vi "Get Path Data.vi"(8 "error in":errorcluster, 11 "Path":path) -> (0 "error out":errorcluster, 3 "Path stuff":T4 {"output cluster"."Limits"."StoopidFast (fps)" min=0.0; "output cluster"."Limits"."Jerk (fps^3)" min=0.0 step=1.0; "output cluster"."Limits"."Accel (fps^2)" min=0.0; "output cluster"."Limits"."Velocity (fps)" min=0.0})   [LabVIEW 2019]
uses:
  Single Cmd Info.ctl
  <vilib>/picture/picture.llb/imagedata.ctl
  types/Limits.ctl
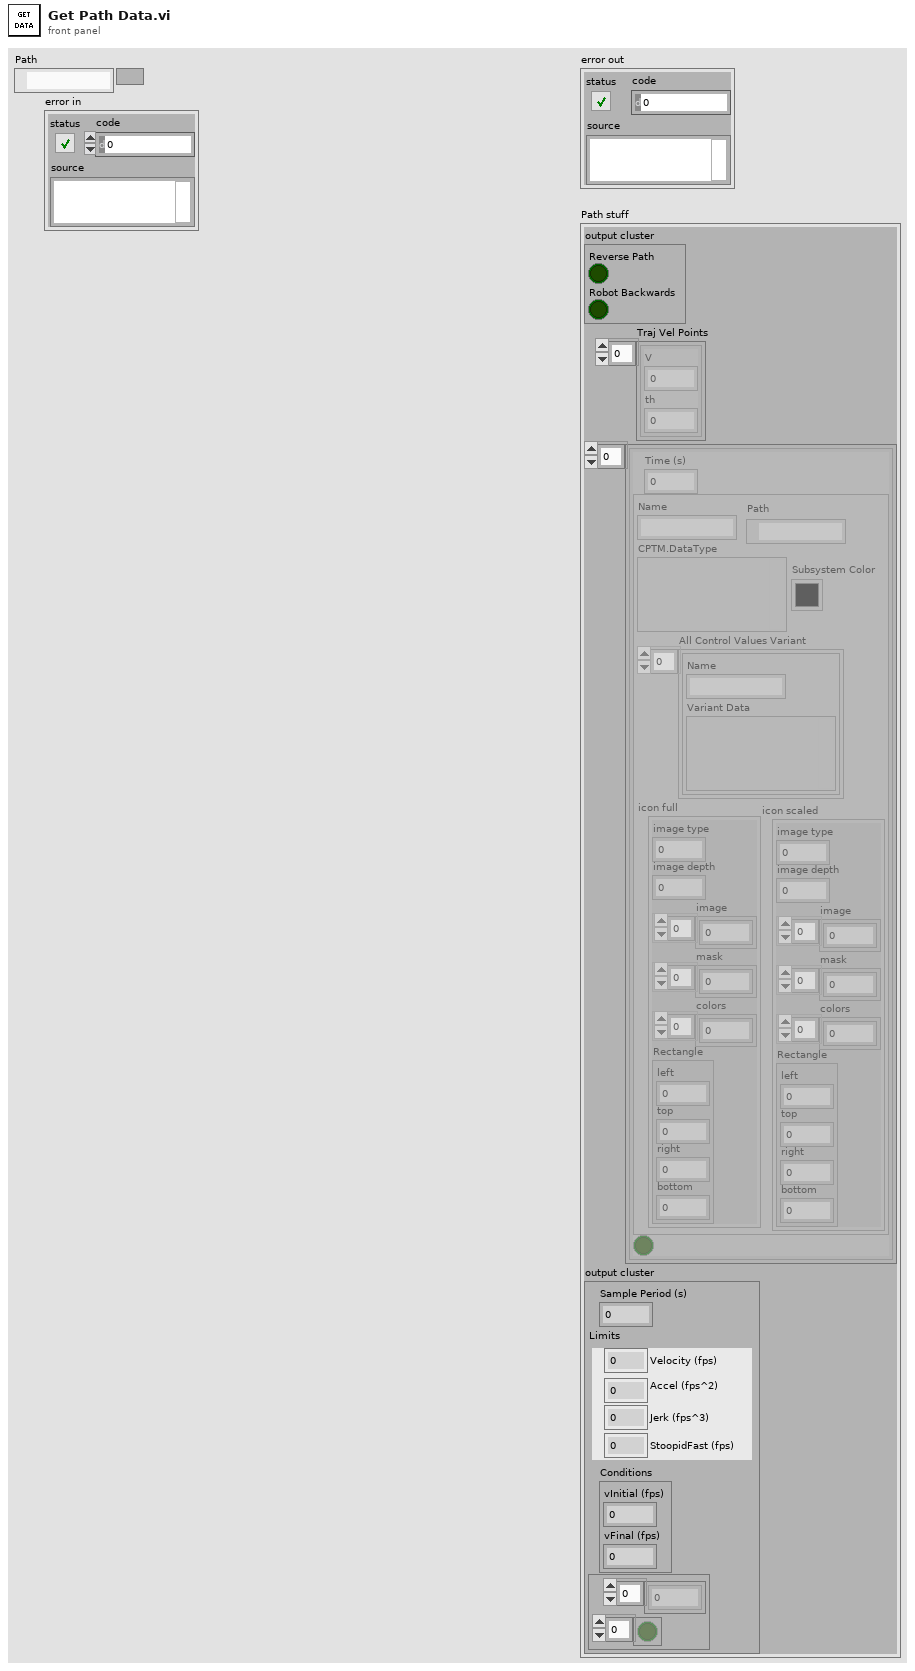
[diagram p1: front panel]
types:
  T1 = typedef "Single Cmd Info.ctl" = cluster{"Name":string, "CPTM.DataType":variant, "All Control Values Variant":cluster{"Name":string, "Variant Data":variant}[], "icon full":T2, "icon scaled":T2, "Path":path, "Subsystem Color":u32}
  T2 = typedef "imagedata.ctl" = cluster{"image type":i32, "image depth":i32, "image":u8[], "mask":u8[], "colors":u32[], "Rectangle":cluster{"left":i16, "top":i16, "right":i16, "bottom":i16}}
  T3 = typedef "Limits.ctl" = cluster{"Velocity (fps)":dbl, "Accel (fps^2)":dbl, "Jerk (fps^3)":dbl, "StoopidFast (fps)":dbl}
  T4 = cluster{"output cluster":cluster{"Reverse Path":bool, "Robot Backwards":bool}, "Traj Vel Points":cluster{"V":dbl, "th":dbl}[], cluster{"Time (s)":dbl, T1, bool}[], "output cluster":cluster{"Sample Period (s)":dbl, "Limits":T3, "Conditions":cluster{"vInitial (fps)":dbl, "vFinal (fps)":dbl}, cluster{dbl[], bool[]}}}
  T5 = cluster{"Segment Name":string, "Type":enum16{"Accel Straight", "Const Straight", "Blend", "Circle"}, "Traj Pos Points":cluster{"x":dbl, "y":dbl, "th":dbl}[], "Traj Vel Points":cluster{"V":dbl, "th":dbl}[], "Accel Index":i32, "Decel Index":i32}[]
  T6 = cluster{"Path Backwards":bool, "Robot Backwards":bool}
  T7 = cluster{"Sample Period (s)":dbl, "Limits":cluster{"Velocity (fps)":dbl, "Acceleration (fps^2)":dbl, "Jerk (fps^3)":dbl}, "Conditions":cluster{"vInitial (fps)":dbl, "vFinal (fps)":dbl}, "Angular Accelerations":cluster{"Angular \nAccelerations":dbl[], "Override Limits?":bool[]}}
  T8 = cluster{"Sample Period (s)":dbl, "Limits":T3, "Conditions":cluster{"vInitial (fps)":dbl, "vFinal (fps)":dbl}, cluster{dbl[], bool[]}}
  T9 = cluster{"Reverse Path":bool, "Robot Backwards":bool}
  T10 = cluster{"Velocity (fps)":dbl, "Acceleration (fps^2)":dbl, "Jerk (fps^3)":dbl}
  T11 = cluster{"vInitial (fps)":dbl, "vFinal (fps)":dbl}
  T12 = cluster{"Angular \nAccelerations":dbl[], "Override Limits?":bool[]}
  T13 = cluster{"Velocity (fps)":dbl, "Acceleration (fps^2)":dbl, "Jerk (fps^3)":dbl, dbl}
  T14 = cluster{"Sample Period (s)":dbl, cluster{"Velocity (fps)":dbl, "Acceleration (fps^2)":dbl, "Jerk (fps^3)":dbl, dbl}, "Conditions":cluster{"vInitial (fps)":dbl, "vFinal (fps)":dbl}, "Angular Accelerations":cluster{"Angular \nAccelerations":dbl[], "Override Limits?":bool[]}}
  T15 = cluster{"Cluster":cluster{"Path Backwards":bool, "Robot Backwards":bool}, "Traj Vel Points":cluster{"V":dbl, "th":dbl}[], cluster{"Time (s)":dbl, T1, bool}[], cluster{"Sample Period (s)":dbl, cluster{"Velocity (fps)":dbl, "Acceleration (fps^2)":dbl, "Jerk (fps^3)":dbl, dbl}, "Conditions":cluster{"vInitial (fps)":dbl, "vFinal (fps)":dbl}, "Angular Accelerations":cluster{"Angular \nAccelerations":dbl[], "Override Limits?":bool[]}}}
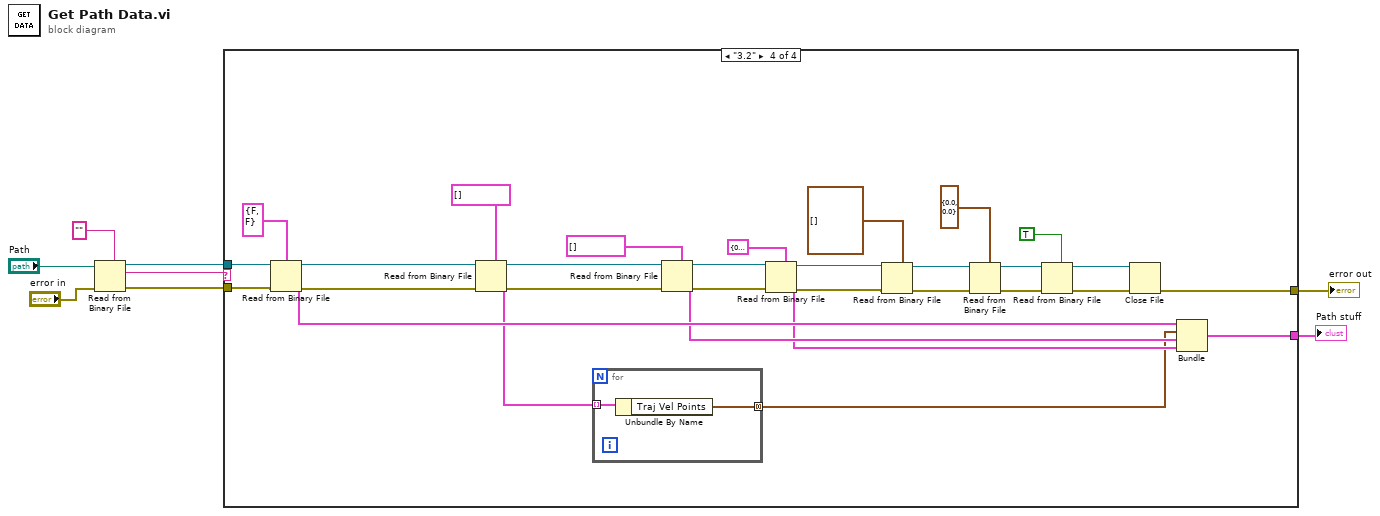
[diagram p0: block diagram]
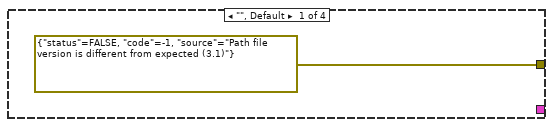
[diagram p2: hidden frame]
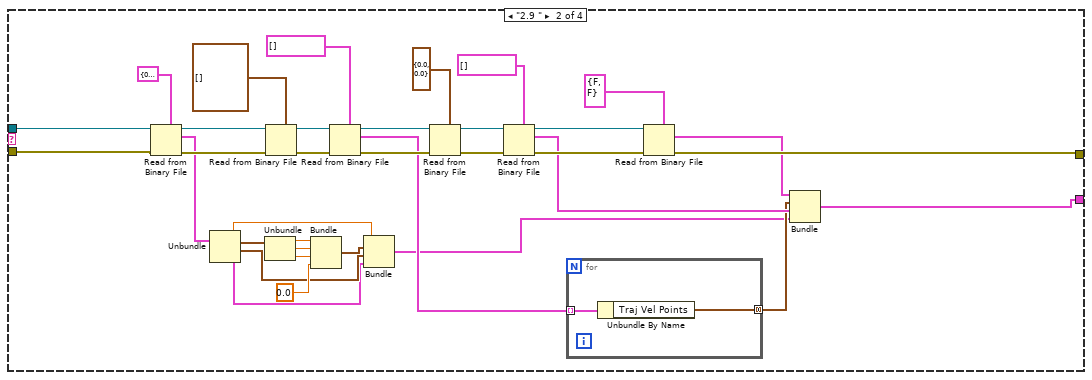
[diagram p3: hidden frame]
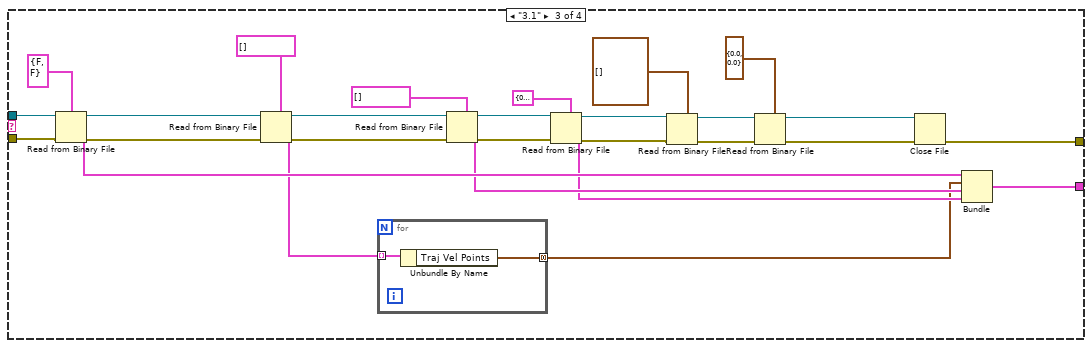
[diagram p4: hidden frame]
diagram:
  n1 = Read from Binary File(5:"", 8:"error in", 11:"Path") -> (0:w4:errorcluster, 2:w2:string, 3:w6:refnum<file>)  [unwired: 3 in, 1 out]
  n2 = case shown="\"3.2\"" w2 {
    tunnel: w6 -> [_ w37 w73 w105]
    tunnel: w4 -> [_ w32 w65 w97]
    tunnel: [errorcluster {"status"=FALSE, "code"=-1, "source"="Path file version is different from expected (3.1)"} ("error out") w26 w53 w87] -> w3
    tunnel: [_ w10 w47 w81] -> w1
    frame "", Default {
    }
    frame "2.9 " {
      n3 = Read from Binary File(5:T7 {"Sample Period (s)"=0.0, "Limits"={"Velocity (fps)"=0.0, "Acceleration (fps^2)"=0.0, "Jerk (fps^3)"=0.0}, "Conditions"={"vInitial (fps)"=0.0, "vFinal (fps)"=0.0}, "Angular Accelerations"={"Angular \nAccelerations"=[], "Override Limits?"=[]}}, 8:w32, 11:w37) -> (0:w31:errorcluster, 2:w21:T7, 3:w40:refnum<file>)  [unwired: 3 in, 1 out]
      n4 = Unbundle(w21) -> ("Sample Period (s)"=w15:dbl, "Limits"=w20:T10, "Conditions"=w13:T11, "Angular Accelerations"=w12:T12)
      n5 = Unbundle(w20) -> ("Velocity (fps)"=w19:dbl, "Acceleration (fps^2)"=w18:dbl, "Jerk (fps^3)"=w17:dbl)
      n6 = Read from Binary File(5:cluster{"x":dbl, "y":dbl, "th":dbl}[] [] ("Points"), 8:w31, 11:w40) -> (0:w30:errorcluster, 3:w41:refnum<file>)  [unwired: 3 in, 2 out]
      n7 = Bundle("Velocity (fps)"=w19, "Acceleration (fps^2)"=w18, "Jerk (fps^3)"=w17, 0.0) -> (w14:T13)  [unwired: 1 in]
      n8 = Read from Binary File(5:T5 [] ("Trajectory Data"), 8:w30, 11:w41) -> (0:w29:errorcluster, 2:w23:T5, 3:w42:refnum<file>)  [unwired: 3 in, 1 out]
      n9 = Bundle("Sample Period (s)"=w15, w14, "Conditions"=w13, "Angular Accelerations"=w12) -> (w11:T14)  [unwired: 1 in]
      n10 = Read from Binary File(5:cluster{"Time (s)":dbl, "Distance (ft)":dbl} {"Time (s)"=0.0, "Distance (ft)"=0.0}, 8:w29, 11:w42) -> (0:w28:errorcluster, 3:w43:refnum<file>)  [unwired: 3 in, 2 out]
      n11 = Read from Binary File(5:cluster{"Time (s)":dbl, T1, bool}[] [], 8:w28, 11:w43) -> (0:w27:errorcluster, 2:w24:cluster{"Time (s)":dbl, T1, bool}[], 3:w44:refnum<file>)  [unwired: 3 in, 1 out]
      n12 = for {
        tunnel: w23 -> [w46] mode=indexing
        tunnel: [w45] -> w22 mode=concatenating
        n13 = Unbundle By Name(w46) -> ("Traj Vel Points"=w45:cluster{"V":dbl, "th":dbl}[])
      }
      n14 = Read from Binary File(5:T6 {"Path Backwards"=FALSE, "Robot Backwards"=FALSE} ("Cluster"), 8:w27, 11:w44) -> (0:w26:errorcluster, 2:w25:T6)  [unwired: 3 in, 2 out]
      n15 = Bundle("Cluster"=w25, "Traj Vel Points"=w22, w24, w11) -> (w10:T15)  [unwired: 1 in]
    }
    frame "3.1" {
      n16 = Read from Binary File(5:T9 {"Reverse Path"=FALSE, "Robot Backwards"=FALSE} ("output cluster"), 8:w65, 11:w73) -> (0:w64:errorcluster, 2:w52:T9, 3:w71:refnum<file>)  [unwired: 3 in, 1 out]
      n17 = Read from Binary File(5:T5 [] ("Trajectory Data"), 8:w64, 11:w71) -> (0:w63:errorcluster, 2:w49:T5, 3:w69:refnum<file>)  [unwired: 3 in, 1 out]
      n18 = for {
        tunnel: w49 -> [w75] mode=indexing
        tunnel: [w74] -> w48 mode=concatenating
        n19 = Unbundle By Name(w75) -> ("Traj Vel Points"=w74:cluster{"V":dbl, "th":dbl}[])
      }
      n20 = Read from Binary File(5:cluster{"Time (s)":dbl, T1, bool}[] [], 8:w63, 11:w69) -> (0:w62:errorcluster, 2:w51:cluster{"Time (s)":dbl, T1, bool}[], 3:w67:refnum<file>)  [unwired: 3 in, 1 out]
      n21 = Read from Binary File(5:T8 {"Sample Period (s)"=0.0, "Limits"={"Velocity (fps)"=0.0, "Accel (fps^2)"=0.0, "Jerk (fps^3)"=0.0, "StoopidFast (fps)"=0.0}, "Conditions"={"vInitial (fps)"=0.0, "vFinal (fps)"=0.0}, {[], []}} ("output cluster"), 8:w62, 11:w67) -> (0:w58:errorcluster, 2:w50:T8, 3:w61:refnum<file>)  [unwired: 3 in, 1 out]
      n22 = Read from Binary File(5:cluster{"x":dbl, "y":dbl, "th":dbl}[] [] ("Updated Waypoints"), 8:w58, 11:w61) -> (0:w57:errorcluster, 3:w59:refnum<file>)  [unwired: 3 in, 2 out]
      n23 = Read from Binary File(5:cluster{"Time (s)":dbl, "Distance (ft)":dbl} {"Time (s)"=0.0, "Distance (ft)"=0.0}, 8:w57, 11:w59) -> (0:w54:errorcluster, 3:w55:refnum<file>)  [unwired: 3 in, 2 out]
      n24 = Close File(refnum=w55, error in=w54) -> (error out=w53:errorcluster)  [unwired: 1 out]
      n25 = Bundle("output cluster"=w52, "Traj Vel Points"=w48, w51, "output cluster"=w50) -> (w47:T4)  [unwired: 1 in]
    }
    frame "3.2" {
      n26 = Read from Binary File(5:T9 {"Reverse Path"=FALSE, "Robot Backwards"=FALSE} ("output cluster"), 8:w97, 11:w105) -> (0:w96:errorcluster, 2:w86:T9, 3:w103:refnum<file>)  [unwired: 3 in, 1 out]
      n27 = Read from Binary File(5:T5 [] ("Trajectory Data"), 8:w96, 11:w103) -> (0:w95:errorcluster, 2:w83:T5, 3:w101:refnum<file>)  [unwired: 3 in, 1 out]
      n28 = for {
        tunnel: w83 -> [w107] mode=indexing
        tunnel: [w106] -> w82 mode=concatenating
        n29 = Unbundle By Name(w107) -> ("Traj Vel Points"=w106:cluster{"V":dbl, "th":dbl}[])
      }
      n30 = Read from Binary File(5:cluster{"Time (s)":dbl, T1, bool}[] [], 8:w95, 11:w101) -> (0:w94:errorcluster, 2:w85:cluster{"Time (s)":dbl, T1, bool}[], 3:w99:refnum<file>)  [unwired: 3 in, 1 out]
      n31 = Read from Binary File(5:T8 {"Sample Period (s)"=0.0, "Limits"={"Velocity (fps)"=0.0, "Accel (fps^2)"=0.0, "Jerk (fps^3)"=0.0, "StoopidFast (fps)"=0.0}, "Conditions"={"vInitial (fps)"=0.0, "vFinal (fps)"=0.0}, {[], []}} ("output cluster"), 8:w94, 11:w99) -> (0:w90:errorcluster, 2:w84:T8, 3:w93:refnum<file>)  [unwired: 3 in, 1 out]
      n32 = Read from Binary File(5:cluster{"x":dbl, "y":dbl, "th":dbl}[] [] ("Updated Waypoints"), 8:w90, 11:w93) -> (0:w89:errorcluster, 3:w91:refnum<file>)  [unwired: 3 in, 2 out]
      n33 = Read from Binary File(5:cluster{"Time (s)":dbl, "Distance (ft)":dbl} {"Time (s)"=0.0, "Distance (ft)"=0.0}, 8:w89, 11:w91) -> (0:w79:errorcluster, 3:w80:refnum<file>)  [unwired: 3 in, 2 out]
      n34 = Read from Binary File(5:TRUE, 8:w79, 11:w80) -> (0:w77:errorcluster, 3:w78:refnum<file>)  [unwired: 3 in, 2 out]
      n35 = Close File(refnum=w78, error in=w77) -> (error out=w87:errorcluster)  [unwired: 1 out]
      n36 = Bundle("output cluster"=w86, "Traj Vel Points"=w82, w85, "output cluster"=w84) -> (w81:T4)  [unwired: 1 in]
    }
  }
  "error out" <- w3
  "Path stuff" <- w1
